vi "Write to TDMS.vi"(8 "error in (no error)":errorcluster, 10 "TDMS File Ref":refnum<k34>, 11 "Logging Data in":refnum<class "Logging Data.lvclass">) -> (0 "error out":errorcluster)   [LabVIEW 2024, in "Logging Data.lvlib" / "Logging Data.lvclass"]
uses:
  Logging Data.lvclass
  Logging Data.lvclass/Logging Data.ctl
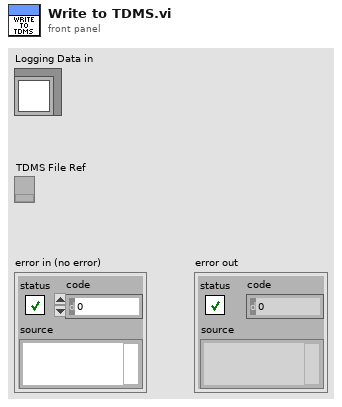
[diagram p1: front panel]
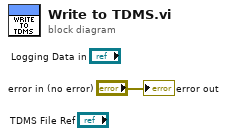
[diagram p0: block diagram]
diagram:
  "error out" <- "error in (no error)"
